vi "Set Installer Destination.vi"(8 "error in":errorcluster, 10 "INST_buildLocation":path=path "C:/testing/testing", 11 ".lvproj":path=path "C:/Users/pauloneill/SCC/Orion/LabVIEW/Source/App/Orion.lvproj") -> (0 "error out":errorcluster)   [LabVIEW 2020, in "CICD.lvlib"]
doc: "Set the Installer Build Location by editing the .LVPROJ XML."
uses:
  CICD.lvlib
  <vilib>/xml/NI_XML.lvlib
  <resource>/objmgr/DOMUserDefRef.rc
  <vilib>/xml/Close Reference(Node).vi
  <vilib>/xml/Load XML File.vi
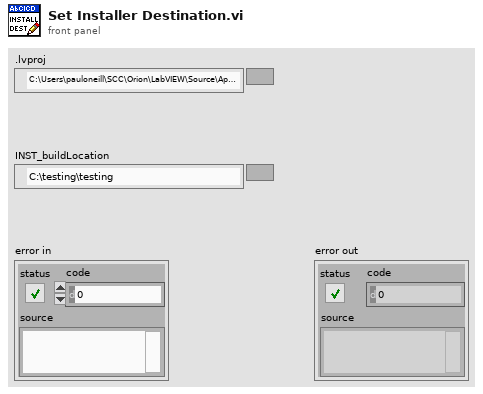
[diagram p1: front panel]
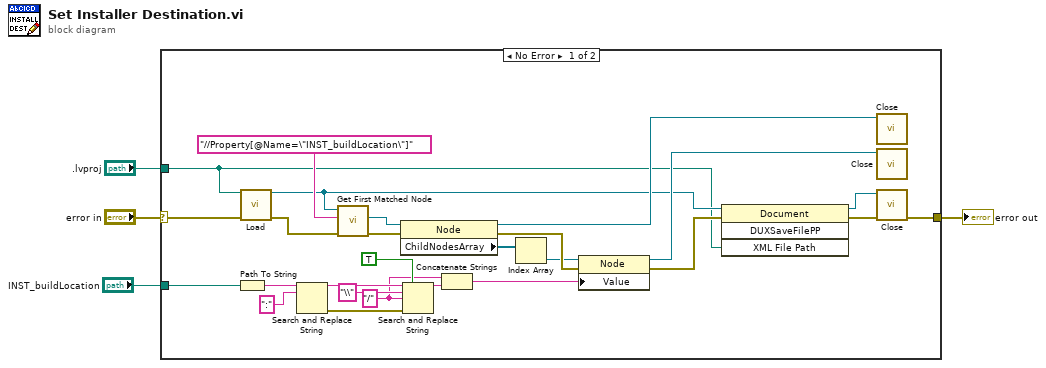
[diagram p0: block diagram]
diagram:
  n1 = case shown="No Error" "error in" {
    selector: "error in" -> [w23 w31]
    tunnel: [w29 w31] -> w4
    tunnel: "INST_buildLocation" -> [w18 _]
    tunnel: ".lvproj" -> [w5 _]
    frame No Error {
      w10 = "/" ("replace string (\"\")")
      n2 = Path To String(path=w18) -> (string=w16:string)
      n3 = call-poly <vilib>:"Load.vi"("path to XML document"=w5, "error in (no error)"=w23) -> ("DOM document out"=w7:refnum<k20>, "error out"=w30:errorcluster)  [unwired: 11 in, 1 out]
      n4 = Search and Replace String(input string=w16, search string=":") -> (result string=w15:string, error out=w26:errorcluster)  [unwired: 6 in, 2 out]
      n5 = call <vilib>:"Get First Matched Node.vi"("error in (no error)"=w30, "XPath expression"="//Property[@Name=\"INST_buildLocation\"]", "node in"=w7) -> ("error out"=w28:errorcluster, "node result"=w20:refnum<k20>)  [unwired: 6 in, 1 out]
      n6 = property class="Node"(reference=w20, error in=w28) -> (reference out=w17:refnum<k20>, error out=w27:errorcluster, "ChildNodesArray"=w21:refnum<k20>[])
      n7 = Search and Replace String(replace all?=TRUE ("replace all? (F)"), input string=w15, search string="\\", replace string=w10, error in=w26) -> (result string=w14:string)  [unwired: 3 in, 3 out]
      n8 = Concatenate Strings(w10, w14) -> (w9:string)
      n9 = Index Array(array=w21) -> (element=w19:refnum<k20>)  [unwired: 1 in]
      n10 = property class="Node"(reference=w19, error in=w27, "Value"=w9) -> (reference out=w8:refnum<k20>, error out=w25:errorcluster)
      n11 = invoke class="Document" method="DUXSaveFilePP"(reference=w7, error in=w25, "XML File Path"=w5) -> (reference out=w6:refnum<k20>, error out=w24:errorcluster)  [unwired: 1 in, 2 out]
      n12 = call-poly <vilib>:"Close.vi"("node"=w17) -> ()  [unwired: 8 in, 1 out]
      n13 = call-poly <vilib>:"Close.vi"("node"=w8) -> ()  [unwired: 8 in, 1 out]
      n14 = call-poly <vilib>:"Close.vi"("error in (no error)"=w24, "node"=w6) -> ("error out"=w29:errorcluster)  [unwired: 7 in]
    }
    frame Error {
    }
  }
  "error out" <- w4
